vi "Open.vi"(8 "error in (no error)":errorcluster, 11 "Shadow in":refnum<class "Shadow.lvclass">) -> (0 "error out":errorcluster, 3 "Shadow out":refnum<class "Shadow.lvclass">)   [LabVIEW 2021, in "UIShadow.lvlib" / "Shadow.lvclass"]
uses:
  Shadow.lvclass
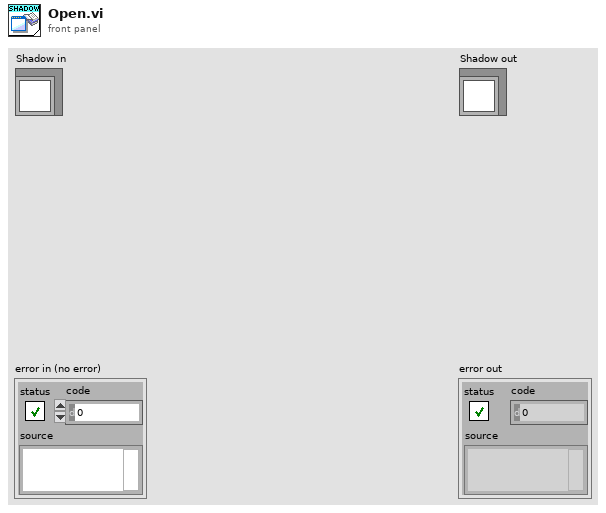
[diagram p1: front panel]
types:
  T1 = enum32{"Invalid", "Standard", "Closed", "Hidden", "Minimized", "Maximized"}
  T2 = typedef "UIShadow.lvlib/Shadow.lvclass/Data.ctl" = cluster{"VI Refnum":refnum<vi>, "ShadowColor":u32, "Offset":i16, "Transparancy":i32, "UIShadowRef":refnum<vi>, "Activate?":bool}
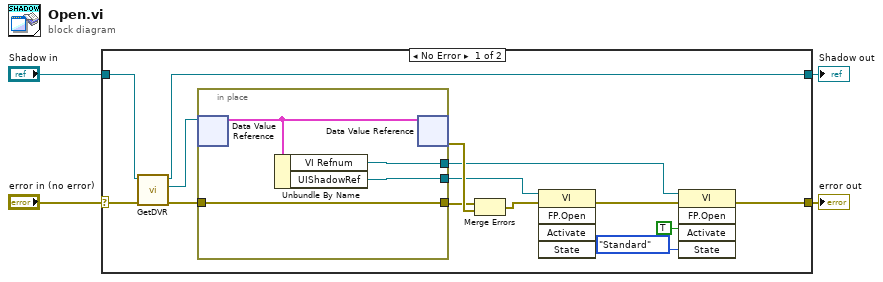
[diagram p0: block diagram]
diagram:
  n1 = case shown="No Error" "error in (no error)" {
    selector: "error in (no error)" -> [w18 w24]
    tunnel: [w8 w24] -> w3
    tunnel: [w17 w23] -> w1
    tunnel: "Shadow in" -> [w16 w23]
    frame No Error {
      n2 = call "GetDVR.vi"("error in (no error)"=w18, "Shadow in"=w16) -> ("error out"=w12:errorcluster, "DVR"=w13:refnum<data-value>, "Shadow out"=w17:refnum<class "Shadow.lvclass">)  [unwired: 7 in]
      n3 = in-place {
        in-place-border: w12 -> [w22]
        in-place-border: [w22] -> w14
        in-place-border: [w20] -> w7
        in-place-border: [w19] -> w10
        n4 = in-place-dvr #1(w13) -> (w21:T2)  [unwired: 1 out]
        n5 = Unbundle By Name(w21) -> ("VI Refnum"=w20:refnum<vi>, "UIShadowRef"=w19:refnum<vi>)
        n6 = in-place-dvr #1(w21) -> (w15:errorcluster)  [unwired: 1 out]
      }
      n7 = Merge Errors(w14, w15) -> (w11:errorcluster)
      n8 = invoke class="VI" method="FP.Open"(reference=w10, error in=w11) -> (error out=w9:errorcluster)  [unwired: 3 in, 4 out]
      n9 = invoke class="VI" method="FP.Open"(reference=w7, error in=w9, "Activate"=TRUE ("Activate?"), "State"=T1."Standard") -> (error out=w8:errorcluster)  [unwired: 1 in, 4 out]
    }
    frame Error {
    }
  }
  "error out" <- w3
  "Shadow out" <- w1
